vi "sub vi - InitializeHysteresisParameters (All axis).vi"(10 "frequency":dbl=0.5) -> ()   [LabVIEW 2010]
panel:
  # "About this Program:\n     - Resets all of the Hysteresis Parameters to\n       values obtained via strain gauge calibration"
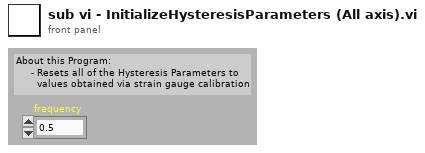
[diagram p1: front panel]
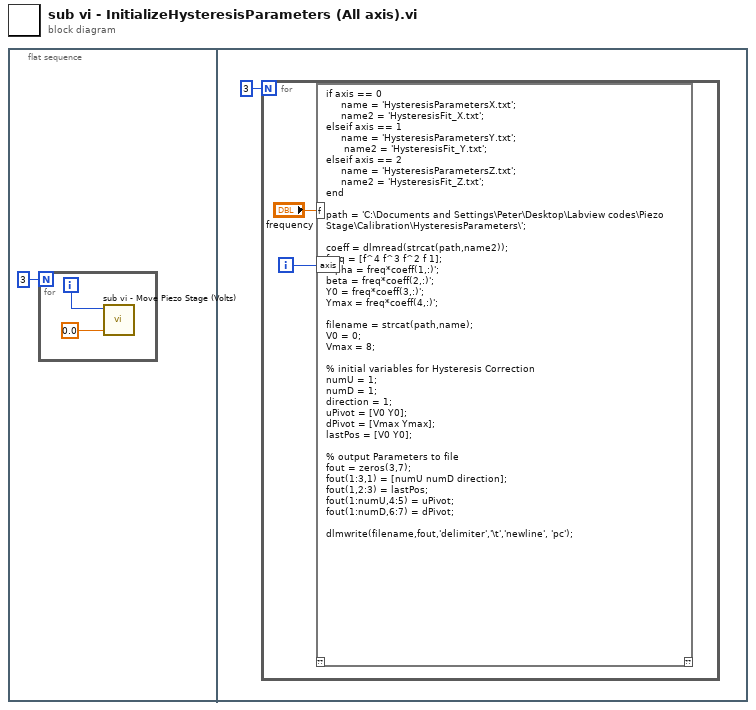
[diagram p0: block diagram]
diagram:
  n1 = flat-sequence {
    frame #0 {
      n2 = for {
        N: 3 -> [_]
        i -> [w2]
        n3 = call "sub vi - Move Piezo Stage (Volts).vi"("Volts"=0.0 ("Desired Position (um)"), "Axis"=w2) -> ()  [unwired: 10 in]
      }
    }
    frame #1 {
      n4 = for {
        N: 3 -> [_]
        i -> [w6]
        n5 = script code="if axis == 0\n     name = 'HysteresisParametersX.txt';\n     name2 = 'HysteresisFit_X.txt';\nelseif axis == 1\n     name = 'HysteresisParametersY.txt';\n      name2 = 'HysteresisFit_Y.txt';\nelseif axis == 2\n     name = 'HysteresisParametersZ.txt';\n     name2 = 'HysteresisFit_Z.txt';\nend\n\npath = 'C:\\Documents and Settings\\Peter\\Desktop\\Labview codes\\Piezo Stage\\Calibration\\HysteresisParameters\\';\n\ncoeff = dlmread(strcat(path,name2));\nfreq = [f^4 f^3 f^2 f 1];\nalpha = freq*coeff(1,:)';\nbeta = freq*coeff(2,:)';\nY0 = freq*coeff(3,:)';\nYmax = freq*coeff(4,:)';\n\nfilename = strcat(path,name);\nV0 = 0;\nVmax = 8;\n\n% initial variables for Hysteresis Correction\nnumU = 1;\nnumD = 1;\ndirection = 1;\nuPivot = [V0 Y0];\ndPivot = [Vmax Ymax];\nlastPos = [V0 Y0];\n\n% output Parameters to file\nfout = zeros(3,7);\nfout(1:3,1) = [numU numD direction];\nfout(1,2:3) = lastPos;\nfout(1:numU,4:5) = uPivot;\nfout(1:numD,6:7) = dPivot;\n     \ndlmwrite(filename,fout,'delimiter','\\t','newline', 'pc');"("axis"=w6, "f"="frequency") -> ()  [unwired: 2 out]
      }
    }
  }
